vi "Jog.vi"(6 "wait for reply (T)":bool=TRUE, 8 "error in":errorcluster, 9 "[rpm]":u16=60, 10 "CCW? (T)":bool=TRUE, 11 "Module ID":i32=-1) -> (0 "error out":errorcluster, 1 "timed out?":bool, 2 "Angle":dbl)   [LabVIEW 2025, in "Stepper.lvlib"]
doc: "_____\nCreated using DQMH Framework: Event Scripter 7.1.2.1547."
uses:
  Stepper.lvlib
  Jog Argument--cluster.ctl
  Jog (Reply Payload)--cluster.ctl
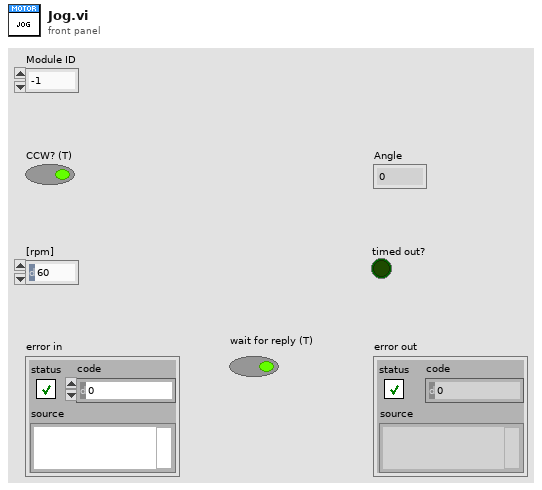
[diagram p1: front panel]
types:
  T1 = typedef "Stepper.lvlib/Jog Argument--cluster.ctl" = cluster{"Module ID":i32, "CCW? (T)":bool, "[rpm]":u16, "Wait Notifier":refnum<notifier>, "wait for reply":bool}
  T2 = typedef "Stepper.lvlib/Request Events--cluster.ctl" = cluster{"Stop Module":refnum<user-event>, "Show Panel":refnum<user-event>, "Hide Panel":refnum<user-event>, "Show Diagram":refnum<user-event>, "Get Module Execution Status":refnum<user-event>, "close":refnum<user-event>, "init":refnum<user-event>, "init driver":refnum<user-event>, "Clear Motor Error":refnum<user-event>, "read config":refnum<user-event>, "Read Angle":refnum<user-event>, "Jog":refnum<user-event>}
  T3 = typedef "Stepper.lvlib/Jog (Reply Payload)--cluster.ctl" = cluster{"Module ID":i32, "Angle":dbl, "error":errorcluster}
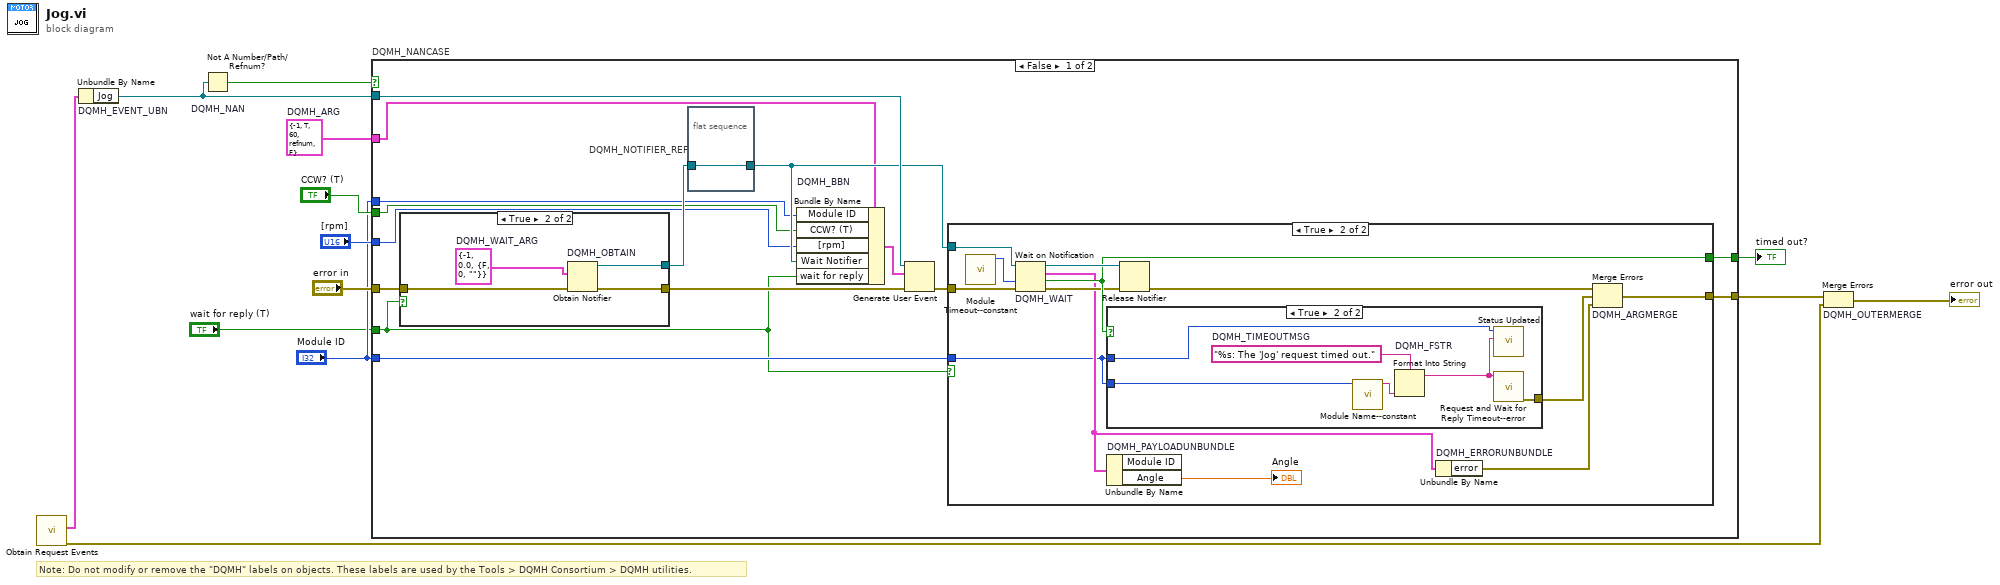
[diagram p0: block diagram]
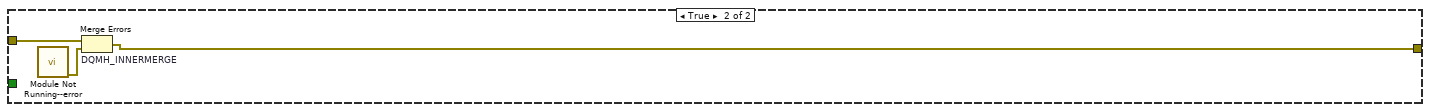
[diagram p5: hidden frame]
diagram:
  w7 = T1 {"Module ID"=-1, "CCW? (T)"=TRUE, "[rpm]"=60, "Wait Notifier"=refnum, "wait for reply"=FALSE}  # DQMH_ARG
  # "Note: Do not modify or remove the \"DQMH\" labels on objects. These labels are used by the Tools > DQMH Consortium > DQMH utilities."
  n1 = call "Obtain Request Events.vi"() -> ("error out"=w2:errorcluster, "Stepper Request Events"=w1:T2)  [unwired: 10 in]
  n2 = Unbundle By Name "DQMH_EVENT_UBN"(w1) -> ("Jog"=w11:refnum<user-event>)
  n3 = Not A Number/Path/Refnum? "DQMH_NAN"(number/path/refnum=w11) -> (NaN/Path/Refnum?=w10:bool)
  n4 = case "DQMH_NANCASE" shown="False" w10 {
    tunnel: "error in" -> [w28 w57]
    tunnel: w11 -> [w26 _]
    tunnel: [w23 w56] -> w8
    tunnel: [w24 _] -> w9
    tunnel: w7 -> [w19 _]
    tunnel: "Module ID" -> [w18 _]
    tunnel: "CCW? (T)" -> [w17 _]
    tunnel: "[rpm]" -> [w16 _]
    tunnel: "Module ID" -> [w15 _]
    tunnel: "wait for reply (T)" -> [w14 _]
    frame False {
      n5 = case shown="True" w14 {
        tunnel: w28 -> [w50 w54]
        tunnel: [w50 w53] -> w25
        tunnel: [_ w51] -> w21
        frame False {
        }
        frame True {
          w52 = T3 {"Module ID"=-1, "Angle"=0.0, "error"={"status"=FALSE, "code"=0, "source"=""}}  # DQMH_WAIT_ARG
          n6 = Obtain Notifier "DQMH_OBTAIN"(notification data type=w52, error in (no error)=w54) -> (notifier out=w51:refnum<notifier>, error out=w53:errorcluster)  [unwired: 2 in, 1 out]
        }
      }
      n7 = flat-sequence "DQMH_NOTIFIER_REF" {
        tunnel: w21 -> [w29]
        tunnel: [w29] -> w20
        frame #0 {
        }
      }
      n8 = Bundle By Name "DQMH_BBN"(cluster=w19, "Module ID"=w18, "CCW? (T)"=w17, "[rpm]"=w16, "Wait Notifier"=w20, "wait for reply"=w14) -> (w22:T1)
      n9 = Generate User Event(user event=w26, event data cluster=w22, error in=w25) -> (error out=w27:errorcluster)  [unwired: 1 in, 1 out]
      n10 = case shown="True" w14 {
        tunnel: w27 -> [w30 w43]
        tunnel: w20 -> [_ w42]
        tunnel: [_ w40] -> w24
        tunnel: [w30 w39] -> w23
        tunnel: w15 -> [_ w31]
        frame False {
        }
        frame True {
          n11 = call "Module Timeout--constant.vi"() -> ("Module Timeout"=w33:i32)  [unwired: 11 in]
          n12 = Wait on Notification "DQMH_WAIT"(notifier=w42, timeout in ms (-1)=w33, error in (no error)=w43) -> (notifier out=w41:refnum<notifier>, notification=w34:T3, timed out?=w40:bool, error out=w38:errorcluster)  [unwired: 1 in]
          n13 = case shown="True" w40 {
            tunnel: [_ w47] -> w35
            tunnel: w31 -> [_ w45]
            tunnel: w31 -> [_ w44]
            frame False {
            }
            frame True {
              w49 = "%s: The 'Jog' request timed out."  # DQMH_TIMEOUTMSG
              n14 = call "Module Name--constant.vi"("Module ID"=w44) -> ("Module Name"=w46:string)  [unwired: 10 in]
              n15 = Format Into String "DQMH_FSTR"(format string=w49, w46) -> (resulting string=w48:string)  [unwired: 2 in, 1 out]
              n16 = call "Status Updated.vi"("Status"=w48, "Module ID"=w45) -> ()  [unwired: 9 in, 1 out]
              n17 = call "Request and Wait for Reply Timeout--error.vi"("Error Message"=w48) -> ("error out"=w47:errorcluster)  [unwired: 10 in]
            }
          }
          n18 = Unbundle By Name "DQMH_PAYLOADUNBUNDLE"(w34) -> ("Angle"=→"Angle":dbl)  [unwired: 1 out]
          n19 = Release Notifier(notifier=w41, error in (no error)=w38) -> (error out=w37:errorcluster)  [unwired: 1 in, 2 out]
          n20 = Unbundle By Name "DQMH_ERRORUNBUNDLE"(w34) -> ("error"=w36:errorcluster)
          n21 = Merge Errors "DQMH_ARGMERGE"(w37, w35, w36) -> (w39:errorcluster)
        }
      }
    }
    frame True {
      n22 = call "Module Not Running--error.vi"() -> ("error out"=w55:errorcluster)  [unwired: 11 in]
      n23 = Merge Errors "DQMH_INNERMERGE"(w57, w55) -> (w56:errorcluster)
    }
  }
  "timed out?" <- w9
  n24 = Merge Errors "DQMH_OUTERMERGE"(w8, w2) -> (→"error out":errorcluster)
